vi "Main Host.vi"() -> ()   [LabVIEW 2018]
uses:
  Host Messages.ctl
  Target Telemetry Cluster.ctl
  Target Sensors.ctl
  <vilib>/Utility/Variable/NI_VariableUtilities.lvlib
panel:
  out "Period (uS)":i64
  out "Encoder Angle":dbl(graph)
  in  "Stop":bool
  out "Data Logging":bool
  in  "Log Data":bool
  in  "Confirm File Name":bool
  in  "File Name":string
  out "Cable Force":dbl(graph)
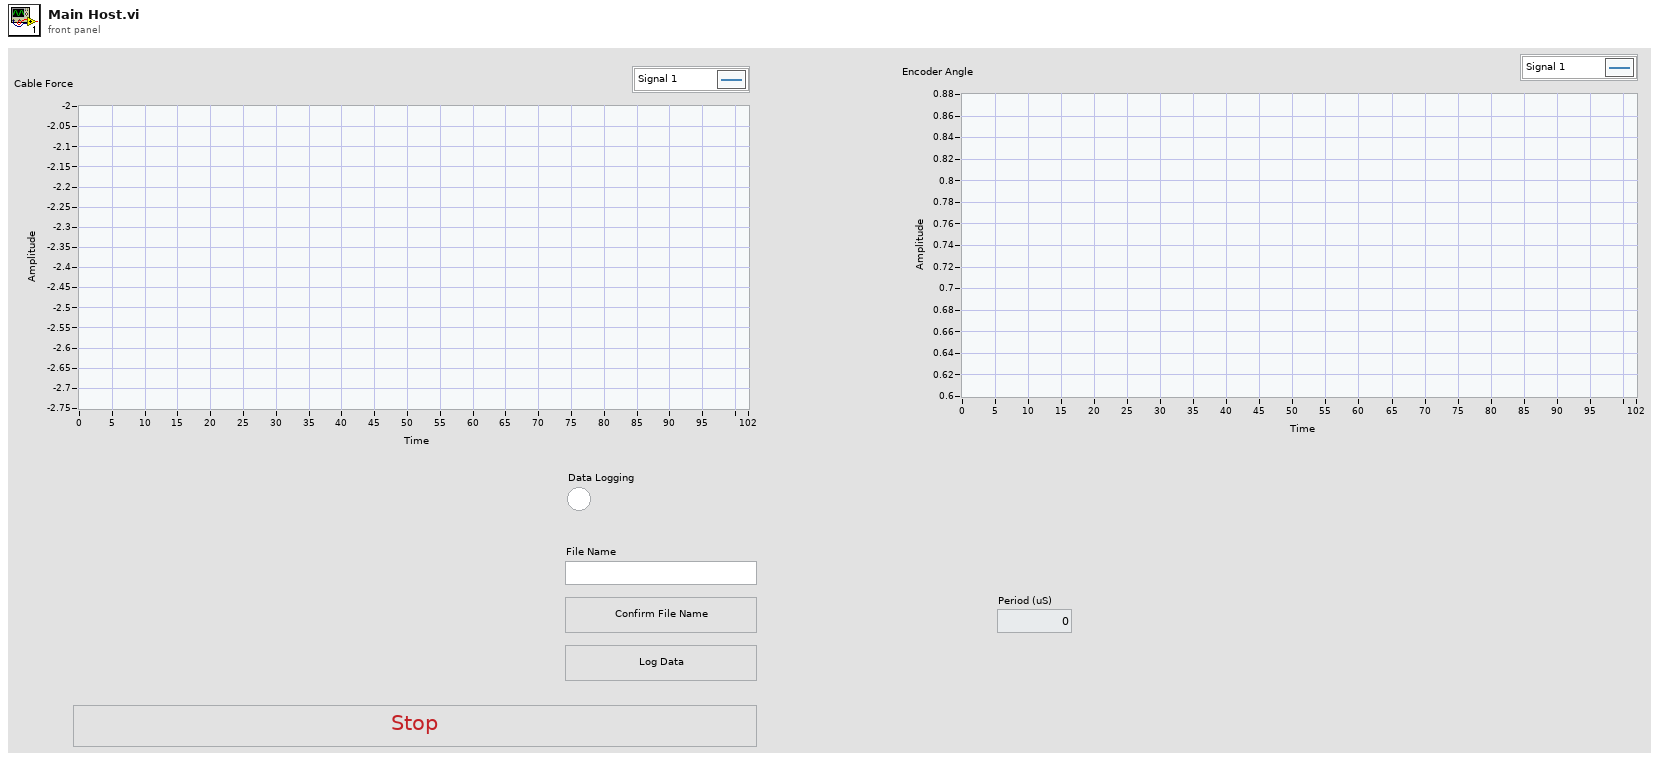
[diagram p1: front panel]
types:
  T1 = typedef "Host Messages.ctl" = enum16{"Stop", "Log Data", "Confirm File Name"}
  T2 = typedef "Target Telemetry Cluster.ctl" = cluster{"Target Sensors":T3}
  T3 = typedef "Target Sensors.ctl" = cluster{"Raw Cable Force (N)":dbl, "Prosthesis Angle (deg)":dbl, "Main Clock Line (s)":dbl}
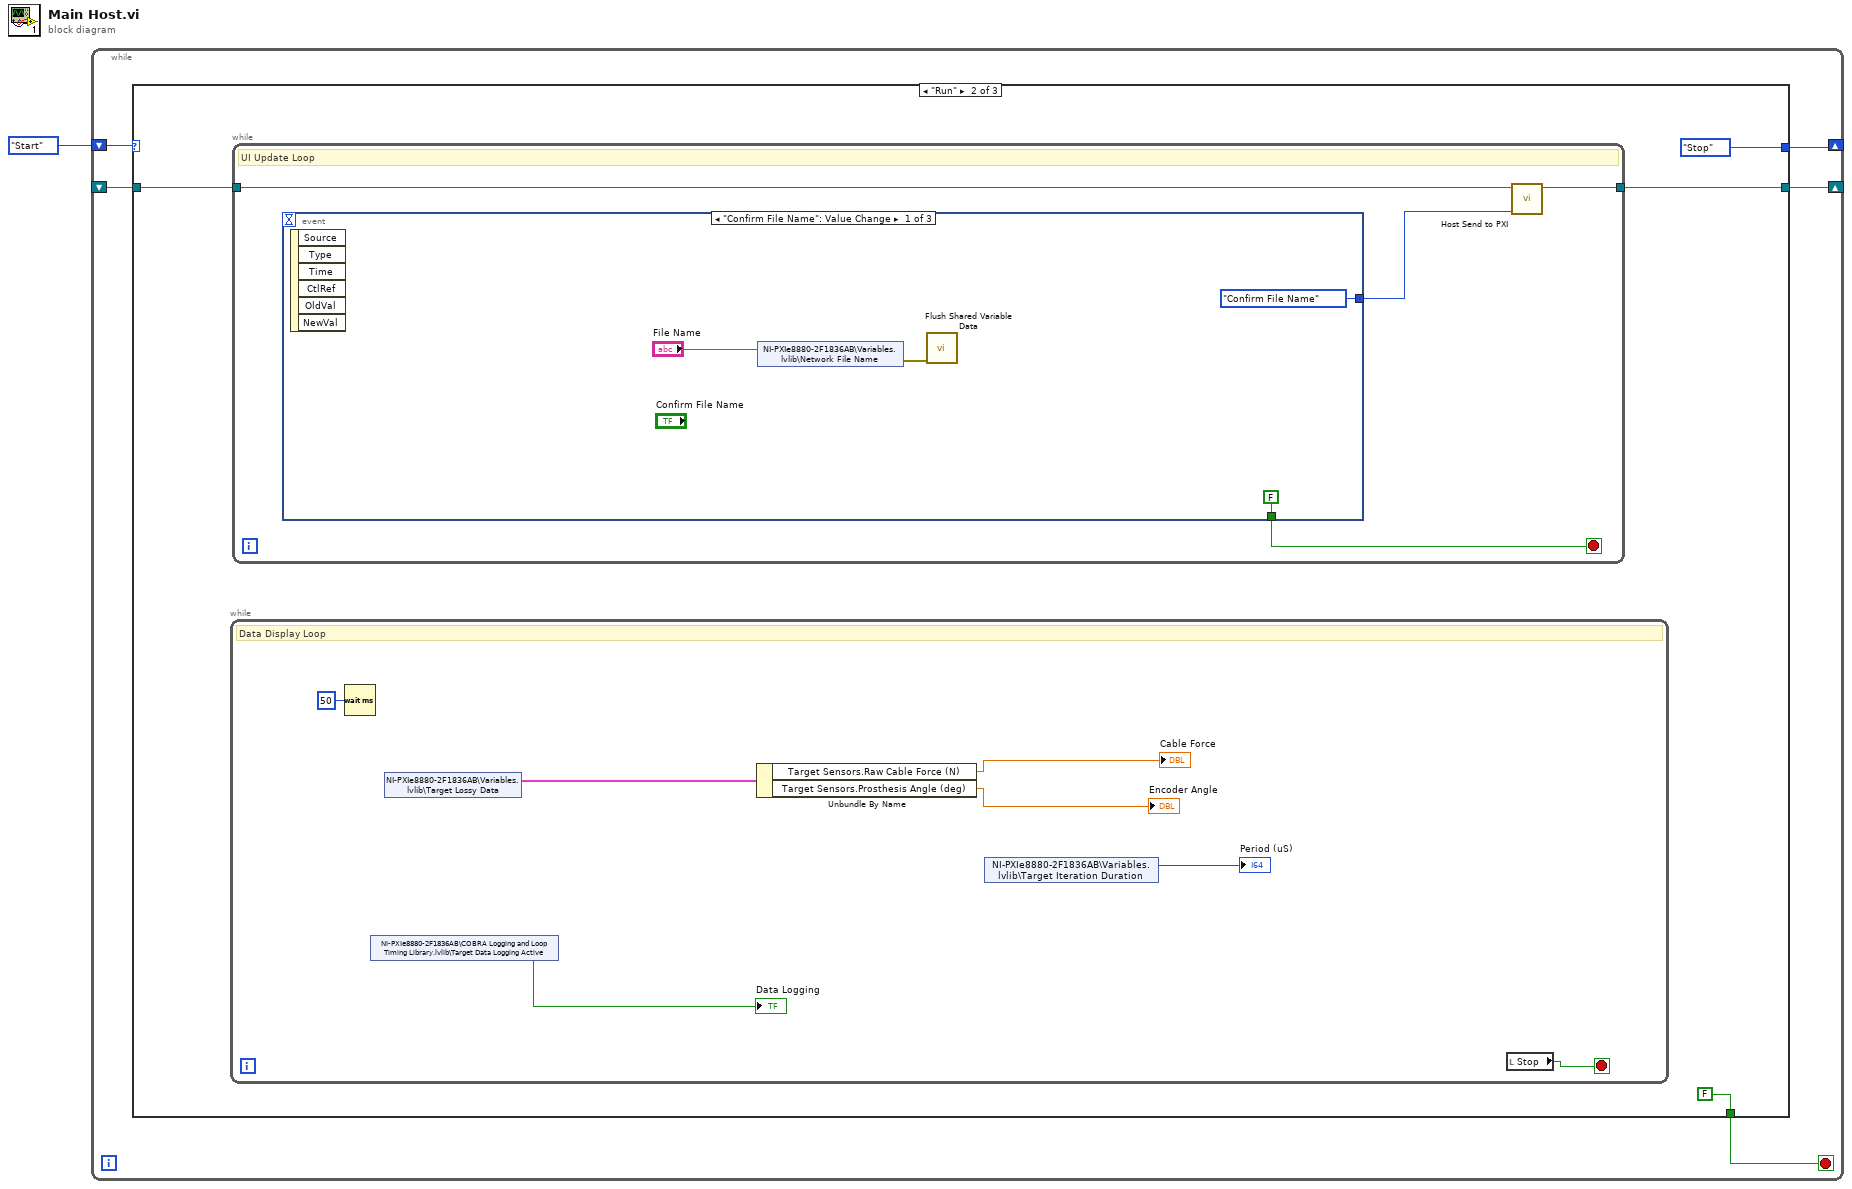
[diagram p0: block diagram]
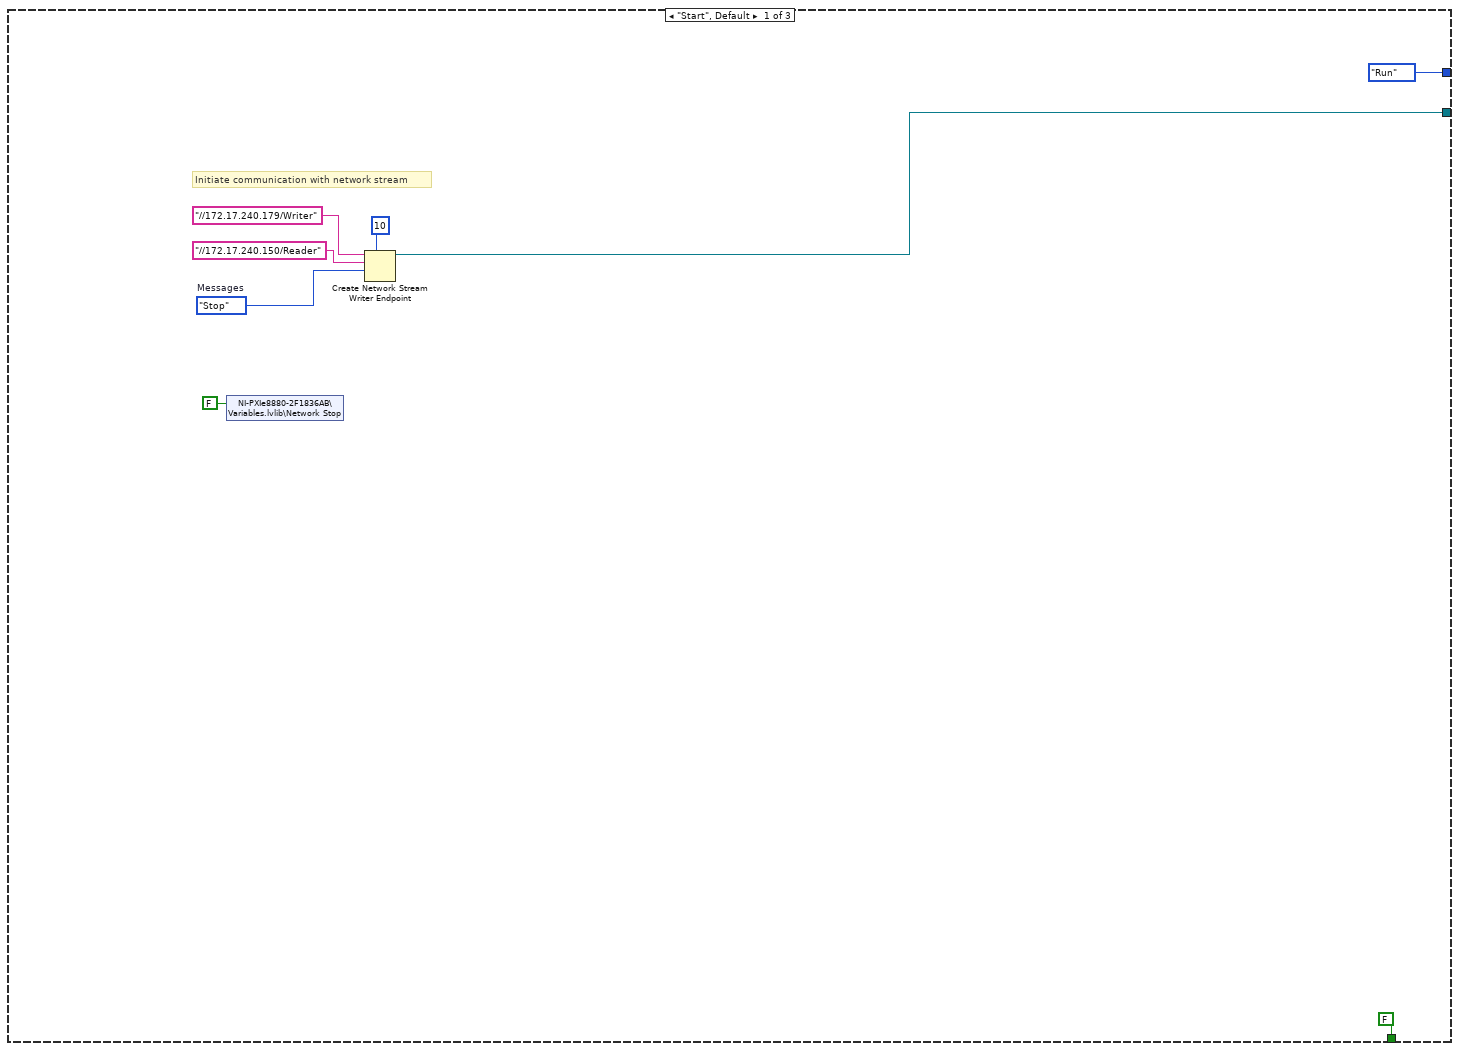
[diagram p2: hidden frame]
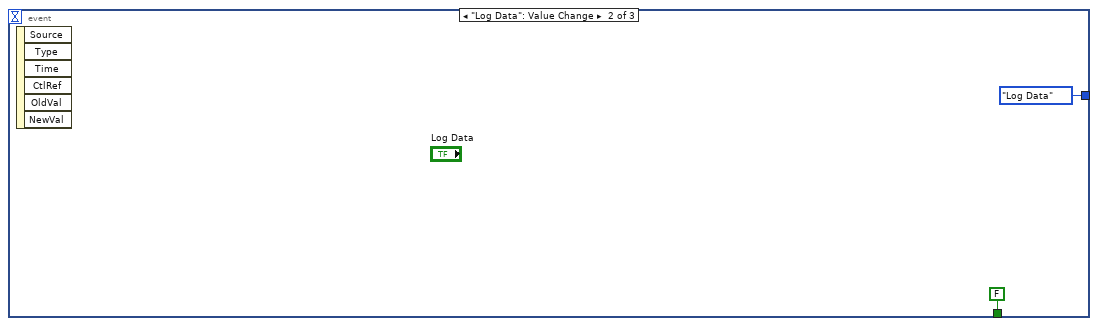
[diagram p3: hidden frame]
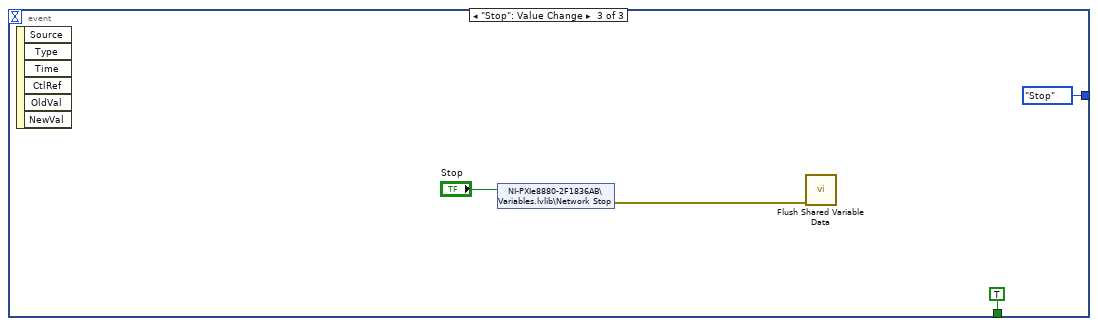
[diagram p4: hidden frame]
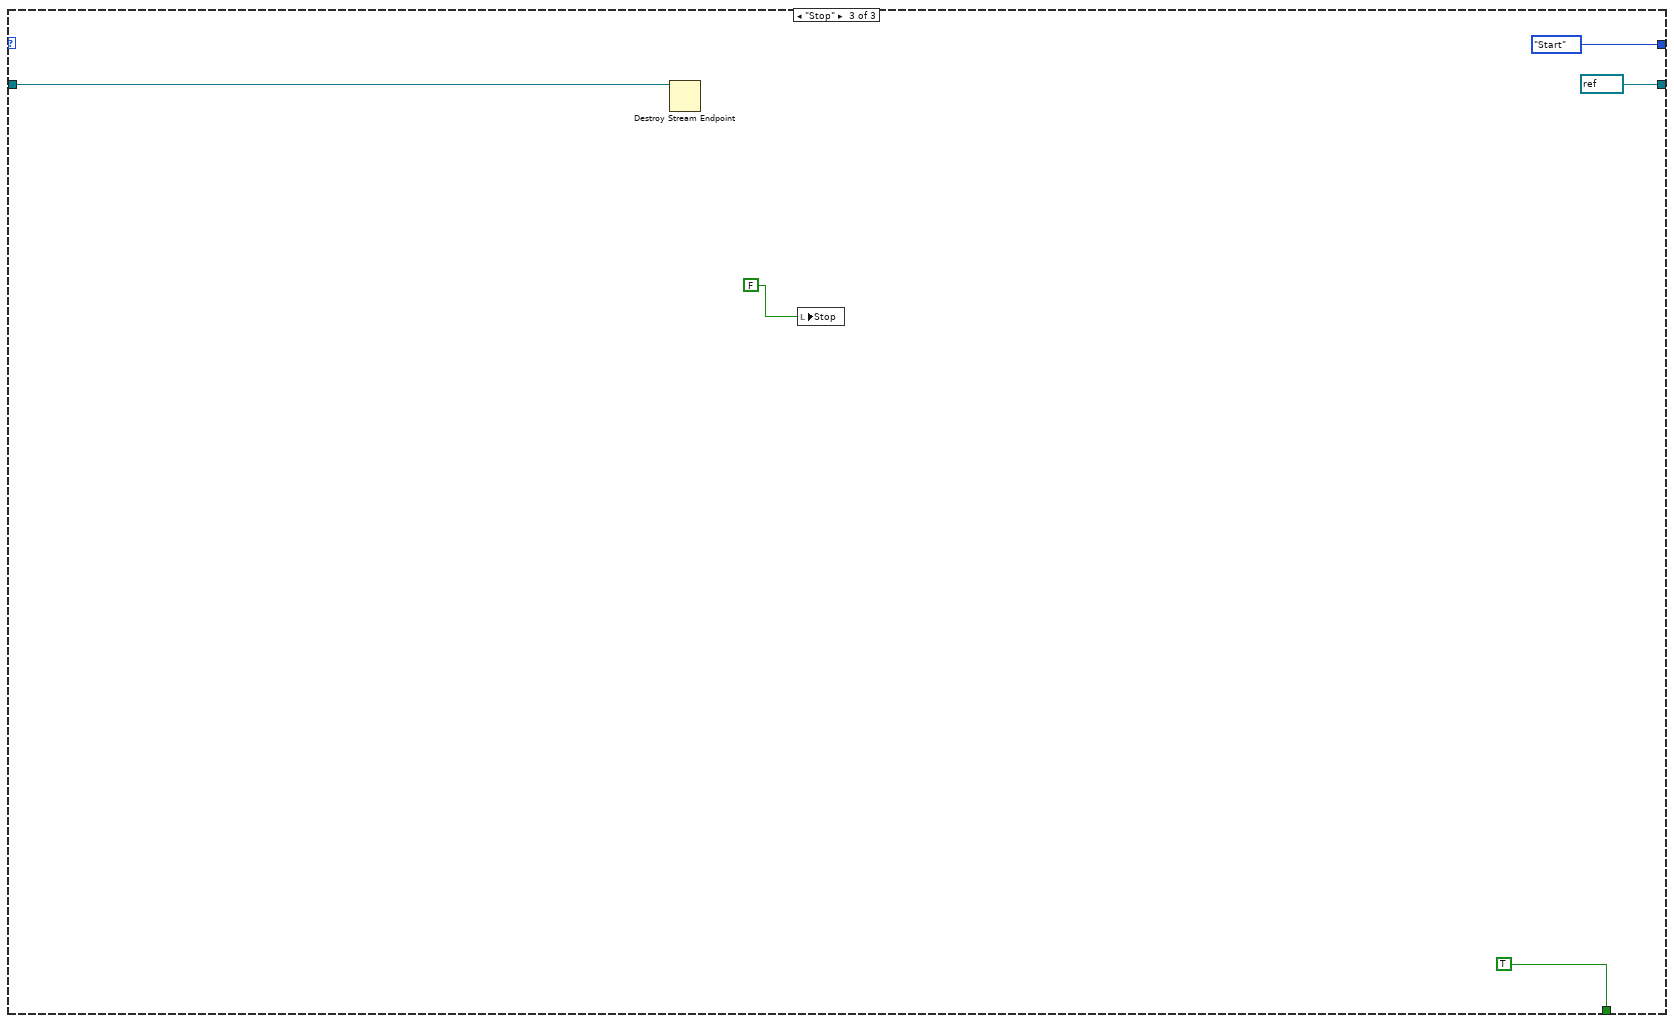
[diagram p5: hidden frame]
diagram:
  n1 = while {
    shift-right: [w5] -> _
    shift-left: enum16{"Start", "Run", "Stop"}."Start" -> [w6]
    shift-right: [w3] -> _
    shift-left: _ -> [w2]
    stop <- w4 stop-if-true
    n2 = case shown="\"Run\"" w6 {
      tunnel: [enum16{"Start", "Run", "Stop"}."Run" enum16{"Start", "Run", "Stop"}."Stop" enum16{"Start", "Run", "Stop"}."Start"] -> w5
      tunnel: [FALSE FALSE TRUE] -> w4
      tunnel: [w9 w15 refnum<k21> refnum ("endpoint out")] -> w3
      tunnel: w2 -> [_ w16 w41]
      frame "Start", Default {
        w8 = Host_Messages."Stop"  # Messages
        # "Initiate communication with network stream"
        n3 = shared-variable "NI-PXIe8880-2F1836AB\\Variables.lvlib\\Network Stop"(FALSE ("Network Stop")) -> ()  [unwired: 1 in, 1 out]
        n4 = Create Network Stream Writer Endpoint(7:10 ("writer buffer size"), 9:w8, 10:"//172.17.240.150/Reader" ("writer name"), 11:"//172.17.240.179/Writer" ("writer name")) -> (3:w9:refnum<k21>)  [unwired: 3 in, 1 out]
      }
      frame "Run" {
        n5 = while {
          stop <- w25 stop-if-true
          # "Data Display Loop"
          n6 = Wait (ms)(milliseconds to wait=u32 50) -> ()  [unwired: 1 out]
          n7 = shared-variable "NI-PXIe8880-2F1836AB\\COBRA Logging and Loop Timing Library.lvlib\\Target Data Logging Active"() -> (→"Data Logging":bool)  [unwired: 1 in, 1 out]
          n8 = shared-variable "NI-PXIe8880-2F1836AB\\Variables.lvlib\\Target Lossy Data"() -> (w22:T2)  [unwired: 1 in, 1 out]
          n9 = Unbundle By Name(w22) -> ("Target Sensors.Raw Cable Force (N)"=→"Cable Force":dbl, "Target Sensors.Prosthesis Angle (deg)"=→"Encoder Angle":dbl)
          n10 = shared-variable "NI-PXIe8880-2F1836AB\\Variables.lvlib\\Target Iteration Duration"() -> (→"Period (uS)":i64)  [unwired: 1 in, 1 out]
          n11 = local read "Stop"() -> (w25:bool)
        }
        n12 = while {
          tunnel: w16 -> [w29]
          tunnel: [w28] -> w15
          stop <- w27 stop-if-true
          # "UI Update Loop"
          n13 = event shown="[0] \"Confirm File Name\": Value Change" {
            selector: _ -> [_ _ _]
            dyn-events: _ -> [_ _ _]
            timeout: _ -> [_ _ _]
            tunnel: [FALSE FALSE TRUE] -> w27
            tunnel: [Host_Messages."Confirm File Name" ("Messages") Host_Messages."Log Data" ("Messages") Host_Messages."Stop" ("Messages")] -> w26
            event "Confirm File Name": Value Change {
              n14 = event-data() -> ()  [unwired: 1 in, 6 out]
              n15 = shared-variable "NI-PXIe8880-2F1836AB\\Variables.lvlib\\Network File Name"("File Name") -> (error out=w30:errorcluster)  [unwired: 1 in]
              n16 = call <vilib>:"Flush Shared Variable Data.vi"("error in (no error)"=w30) -> ()  [unwired: 10 in, 1 out]
            }
            event "Log Data": Value Change {
              n17 = event-data() -> ()  [unwired: 1 in, 6 out]
            }
            event "Stop": Value Change {
              n18 = event-data() -> ()  [unwired: 1 in, 6 out]
              n19 = shared-variable "NI-PXIe8880-2F1836AB\\Variables.lvlib\\Network Stop"("Stop") -> (error out=w36:errorcluster)  [unwired: 1 in]
              n20 = call <vilib>:"Flush Shared Variable Data.vi"("error in (no error)"=w36) -> ()  [unwired: 10 in, 1 out]
            }
          }
          n21 = call "Host Send to PXI.vi"("Messages"=w26, "endpoint in"=w29) -> ("endpoint out"=w28:refnum<k21>)  [unwired: 9 in]
        }
      }
      frame "Stop" {
        n22 = Destroy Stream Endpoint(11:w41) -> ()  [unwired: 1 in, 1 out]
        n23 = local write "Stop"(FALSE ("Force Tracking Mode")) -> ()
      }
    }
  }
